vi "SS2 Live_Refresh All Parameters.vi"(8 "Error In":errorcluster, 9 "Verbose (T)":bool=TRUE, 11 "VI Refnum in":refnum<vi>) -> (0 "Error Out":errorcluster)   [LabVIEW 2019]
uses:
  SS2 Live_Settings List.ctl
  341269f5-52e1-4f88-b524-c1612519b6ae.vi
panel:
  out "Settings Error Source":T1[](array[typedef])
  in  "SS2 Live Settings List":T1
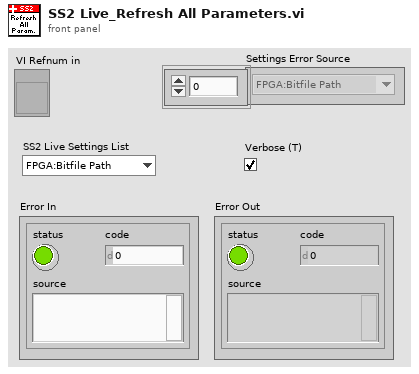
[diagram p1: front panel]
types:
  T1 = typedef "SS2 Live_Settings List.ctl" = enum16{"FPGA:Bitfile Path", "FPGA:Bitfile Version", "FPGA:Auto Reset FPGA", "Acquisition Parameters:SS2 DAQ Parameters", "Acquisition Parameters:Gate Configuration Array", "Acquisition Parameters:Buffer Size (# Gates)", "File Information:File Information", "File Information:# Datasets in Series", "File Information:Scrambled File Flag", "File Information:Delay between Datasets", "Image Parameters:Image ROI Information", "Image Parameters:Image Binning Options", "UI Settings:Histogram Bins Number"}
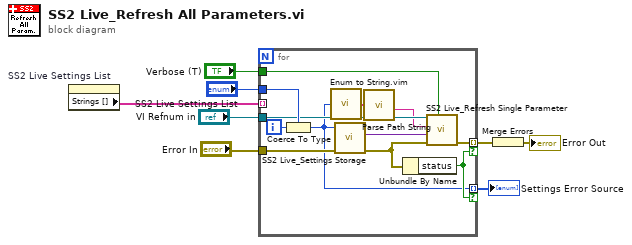
[diagram p0: block diagram]
diagram:
  n1 = property on="SS2 Live Settings List" class="Enum (strict)"() -> ("Strings []"=w6:string[])  [unwired: 2 in, 2 out]
  n2 = for {
    tunnel: "VI Refnum in" -> [w18]
    tunnel: w6 -> [_] mode=indexing
    tunnel: "SS2 Live Settings List" -> [w19]
    tunnel: "Error In" -> [w15]
    tunnel: [w14] -> w4 mode=indexing if=w12
    tunnel: [w10] -> w2 mode=indexing if=w12
    tunnel: "Verbose (T)" -> [w11]
    i -> [w20]
    n3 = Coerce To Type(0:w20, 1:w19) -> (2:w10:T1)
    n4 = call "Enum to String.vim"("Enum"=w10) -> ("String"=w9:string)
    n5 = call "SS2 Live_Settings Storage.vi"("Error In"=w15, "Settings List"=w10) -> ("Error Out"=w13:errorcluster, "Variant Data out"=w16:variant)  [unwired: 8 in]
    n6 = call "Parse Path String.vi"("Path in"=w9) -> ("File/Folder"=w17:string)  [unwired: 4 in, 1 out]
    n7 = Unbundle By Name(w13) -> ("status"=w12:bool)
    n8 = call "SS2 Live_Refresh Single Parameter.vi"("Verbose (T)"=w11, "Error In"=w13, "Data"=w16, "Control Label"=w17, "VI Ref in"=w18) -> ("Error Out"=w14:errorcluster)  [unwired: 6 in]
  }
  "Settings Error Source" <- w2
  n9 = Merge Errors(w4) -> (→"Error Out":errorcluster)
